vi "Write Path.vi"(7 "key":string, 8 "error in (no error)":errorcluster, 9 "default value":path, 10 "refnum":T1, 11 "Process in":refnum<class "Process.lvclass">) -> (0 "error out":errorcluster, 2 "refnum out":T1, 3 "Process out":refnum<class "Process.lvclass">)   [LabVIEW 2020, in "Configuration File.lvlib"]
doc: "High-level function for writing configuration file data from process class."
uses:
  Configuration File.lvlib
  Process Classes/Process/Process.lvclass
  <vilib>/Utility/config.llb/NI_LVConfig.lvlib
  <vilib>/Utility/config.llb/Write Key (Path).vi
  <vilib>/Utility/config.llb/Config Data RefNum.ctl
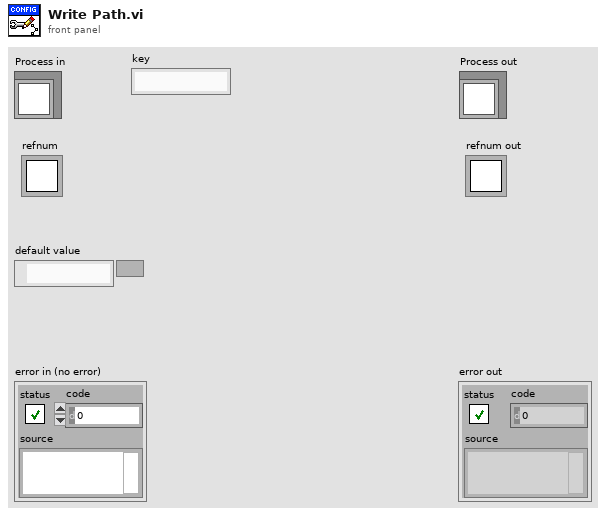
[diagram p1: front panel]
types:
  T1 = typedef "NI_LVConfig.lvlib/Config Data RefNum.ctl" = refnum<k1>
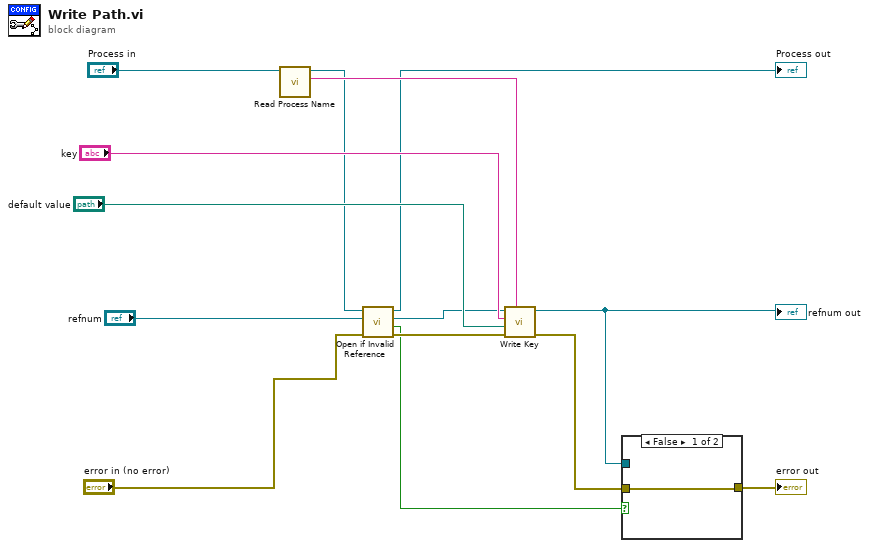
[diagram p0: block diagram]
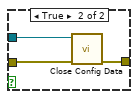
[diagram p2: hidden frame]
diagram:
  n1 = call "Read Process Name.vi"("Process In"="Process in") -> ("Process Name"=w12:string, "Process Out"=w6:refnum<class "Process.lvclass">)  [unwired: 9 in]
  n2 = call "Open if Invalid Reference.vi"("error in (no error)"="error in (no error)", "refnum"="refnum", "Process in"=w6) -> ("error out"=w9:errorcluster, "File opened?"=w2:bool, "refnum out"=w10:T1, "Process out"=→"Process out":refnum<class "Process.lvclass">)  [unwired: 5 in]
  n3 = call-poly <vilib>:"Write Key.vi"("section"=w12, "error in (no error)"=w9, "value"="default value", "key"="key", "refnum"=w10) -> ("error out"=w4:errorcluster, "refnum out"=w5:T1)  [unwired: 4 in, 1 out]
  "refnum out" <- w5
  n4 = case shown="False" w2 {
    tunnel: w5 -> [_ w18]
    tunnel: w4 -> [w15 w17]
    tunnel: [w15 w16] -> w3
    frame False {
    }
    frame True {
      n5 = call <vilib>:"Close Config Data.vi"("error in (no error)"=w17, "refnum"=w18) -> ("error out"=w16:errorcluster)  [unwired: 8 in, 1 out]
    }
  }
  "error out" <- w3
